vi "Write VI Refnum.vi"(8 "error in (no error)":errorcluster, 10 "VI Refnum":refnum<vi>, 11 "UI-Bus_Boolean in":refnum<class "UI-Bus_Single.lvclass">) -> (0 "error out":errorcluster, 3 "UI-Bus_Boolean out":refnum<class "UI-Bus_Single.lvclass">)   [LabVIEW 2021, in "UI-Bus_Single.lvclass"]
uses:
  UI-Bus_Single.lvclass
  UI-Bus_Single.lvclass/UI-Bus_Single.ctl
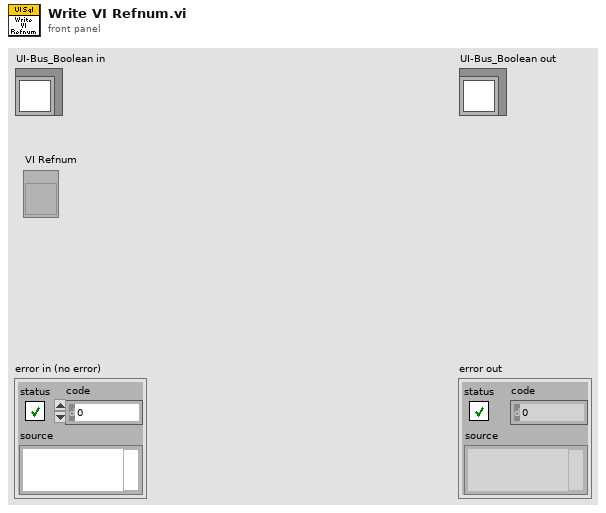
[diagram p1: front panel]
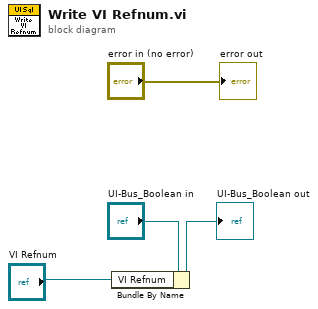
[diagram p0: block diagram]
diagram:
  n1 = Bundle By Name(cluster="UI-Bus_Boolean in", "VI Refnum"="VI Refnum") -> (→"UI-Bus_Boolean out":refnum<class "UI-Bus_Single.lvclass">)
  "error out" <- "error in (no error)"
